vi "Send Notification.vi"(8 "error in":errorcluster, 10 "IMessagePayload.lvclass":refnum<class "IMessagePayload.lvclass">, 11 "NotifierMessageTransport in":refnum<class "NotifierMessageTransport.lvclass">) -> (0 "error out":errorcluster, 3 "NotifierMessageTransport out":refnum<class "NotifierMessageTransport.lvclass">)   [LabVIEW 2016, in "NotifierMessageTransport.lvclass"]
uses:
  NotifierMessageTransport.lvclass
  IMessagePayload/IMessagePayload.lvclass
  NotifierMessageTransport.lvclass/NotifierMessageTransport.ctl
panel:
  # "INPUTS"
  # "OUTPUTS"
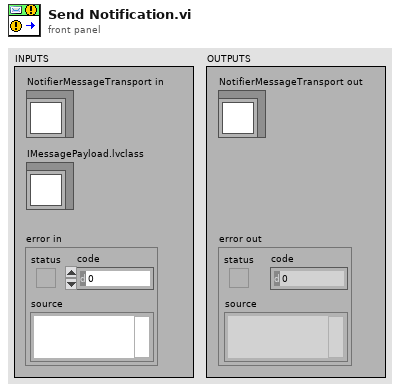
[diagram p1: front panel]
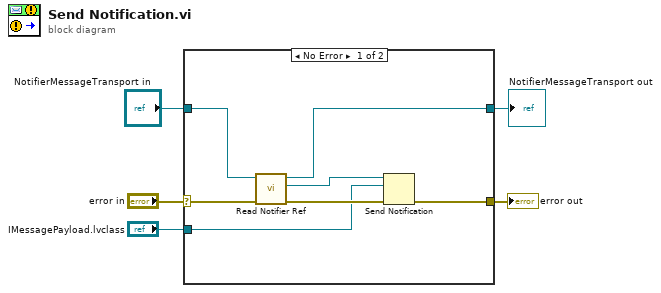
[diagram p0: block diagram]
diagram:
  n1 = case shown="No Error" "error in" {
    selector: "error in" -> [w7 w14]
    tunnel: [w6 w14] -> w4
    tunnel: [w11 w13] -> w1
    tunnel: "NotifierMessageTransport in" -> [w12 w13]
    tunnel: "IMessagePayload.lvclass" -> [w8 _]
    frame No Error {
      n2 = call "Read Notifier Ref.vi"("error in"=w7, "NotifierMessageTransport in"=w12) -> ("error out"=w9:errorcluster, "Notifier Ref"=w10:refnum<notifier>, "NotifierMessageTransport out"=w11:refnum<class "NotifierMessageTransport.lvclass">)  [unwired: 7 in]
      n3 = Send Notification(notification=w8, notifier=w10, error in (no error)=w9) -> (error out=w6:errorcluster)  [unwired: 1 out]
    }
    frame Error {
    }
  }
  "error out" <- w4
  "NotifierMessageTransport out" <- w1
